vi "Get_Coeff_Fr_String.vi"(4 "String Name":string, 5 "Take New Data?":bool, 6 "Prefix":string, 7 "Show Dialog?":bool=TRUE, 8 "Sub String":string, 9 "Inst type":T1=enum."Raw voltage", 10 "Whole String":string) -> (0 "Coefficients Found?":bool, 2 "Calib Constants":dbl[](array[numeric]))   [LabVIEW 2010]
uses:
  Controls/Pressure_Units.ctl
  Controls/Inst_type.ctl
panel:
  in  "Pressure Units":T2
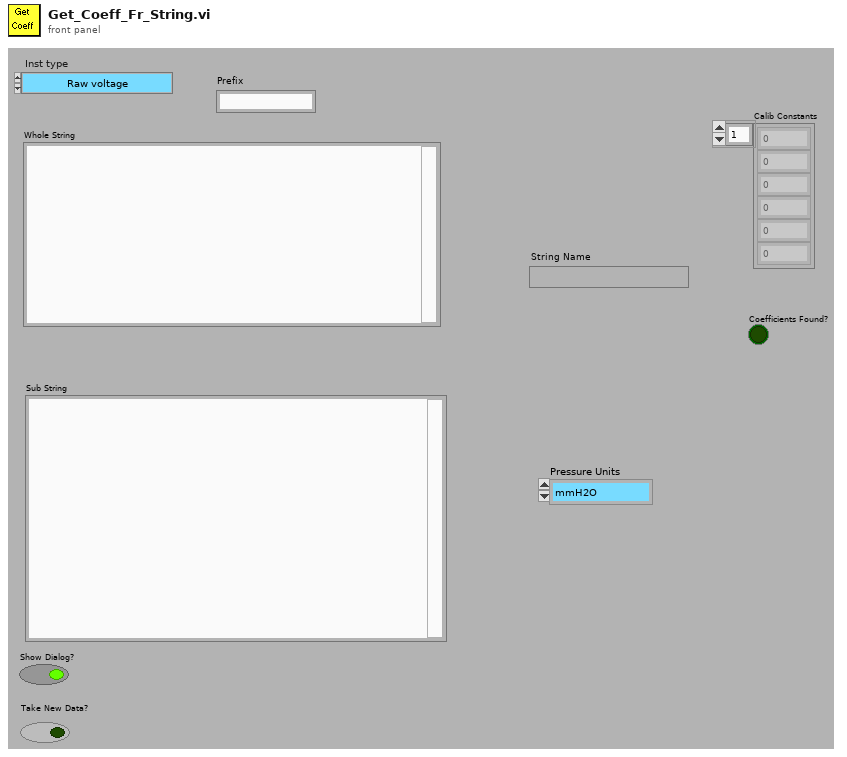
[diagram p1: front panel]
types:
  T1 = typedef "Inst_type.ctl" = enum16{"Propeller anemometer", "Raw voltage", "Pressure Transducer", "Pitot-static tube", "Preston tube", "Hot wire", "Cross wire 1", "Cross wire 2", "Generic Linear", "Generic Polynomial", "Generic BackPoly", "Fast FID", "Thermocouple", "Cold wire", "Pulsed Wire", "LDA Vel", "LDA Tran time", "LDA Arr time"}
  T2 = typedef "Pressure_Units.ctl" = enum16{"mmH2O", "mmHg", "Pa (N/m^2)", "mbar", "bar"}
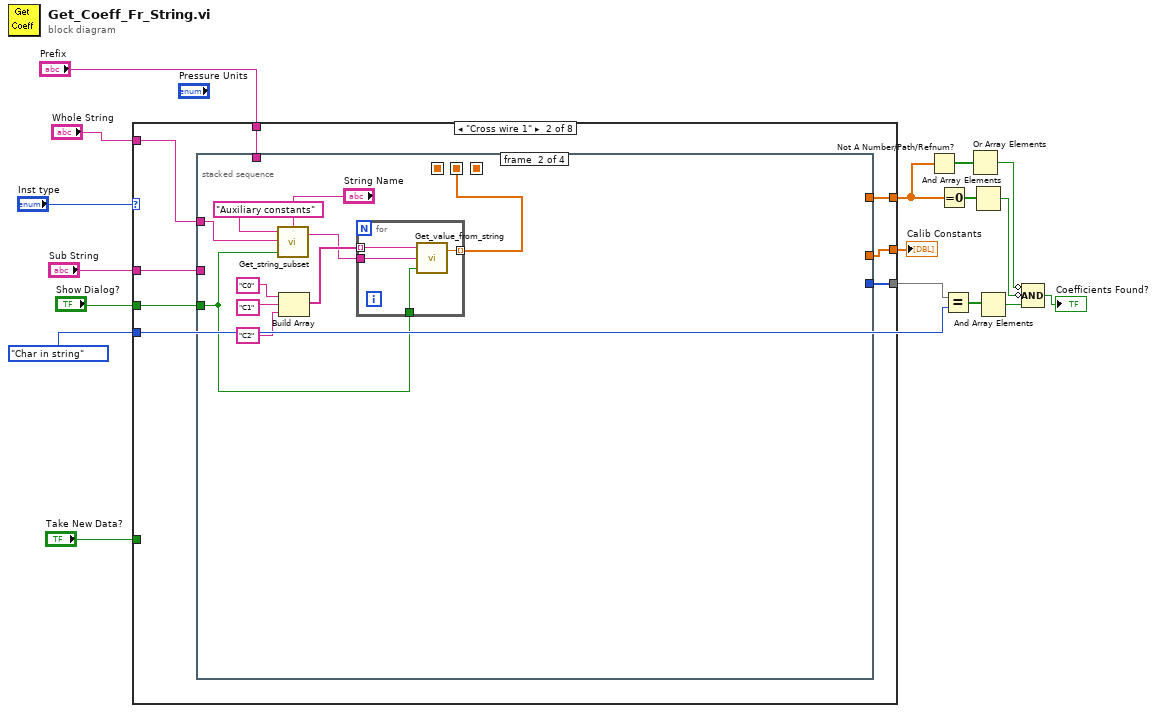
[diagram p0: block diagram]
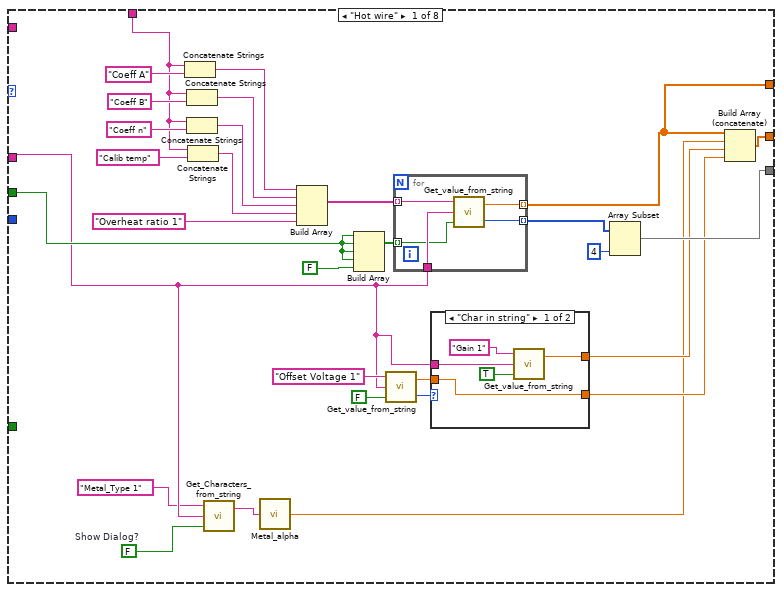
[diagram p2: hidden frame]
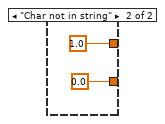
[diagram p3: hidden frame]
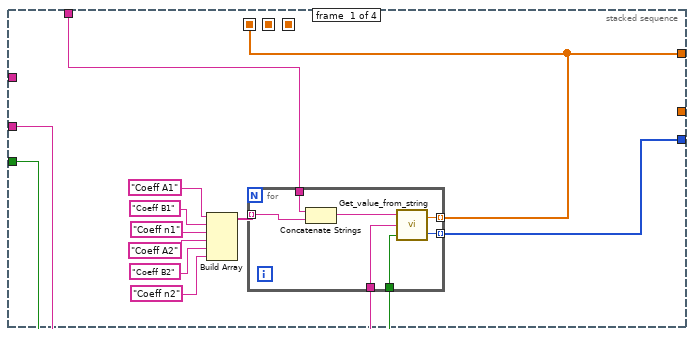
[diagram p4: hidden frame]
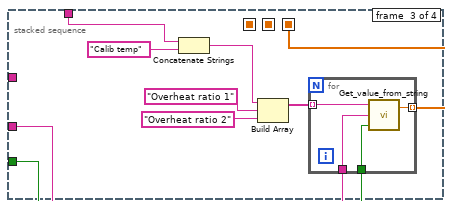
[diagram p5: hidden frame]
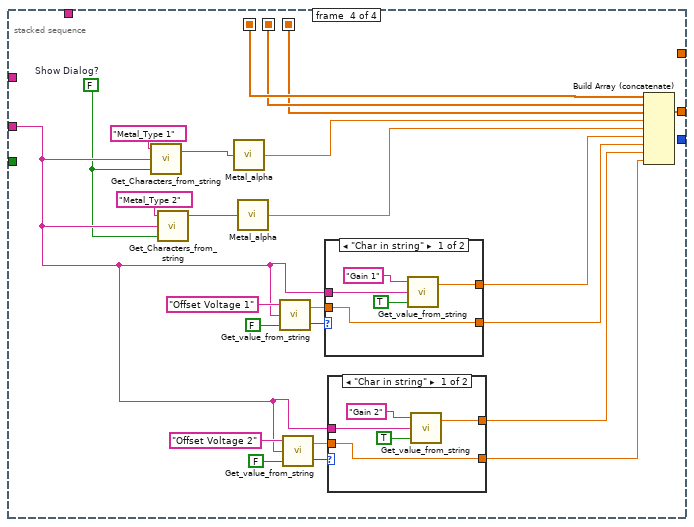
[diagram p6: hidden frame]
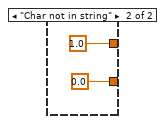
[diagram p7: hidden frame]
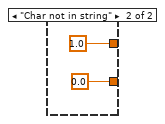
[diagram p8: hidden frame]
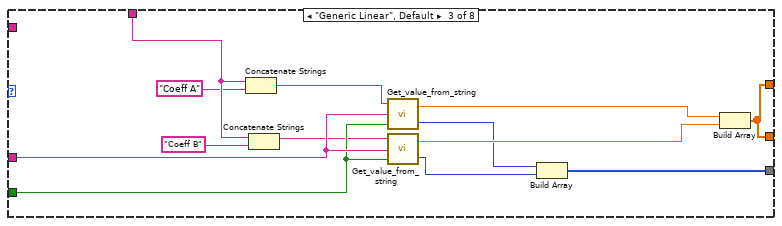
[diagram p9: hidden frame]
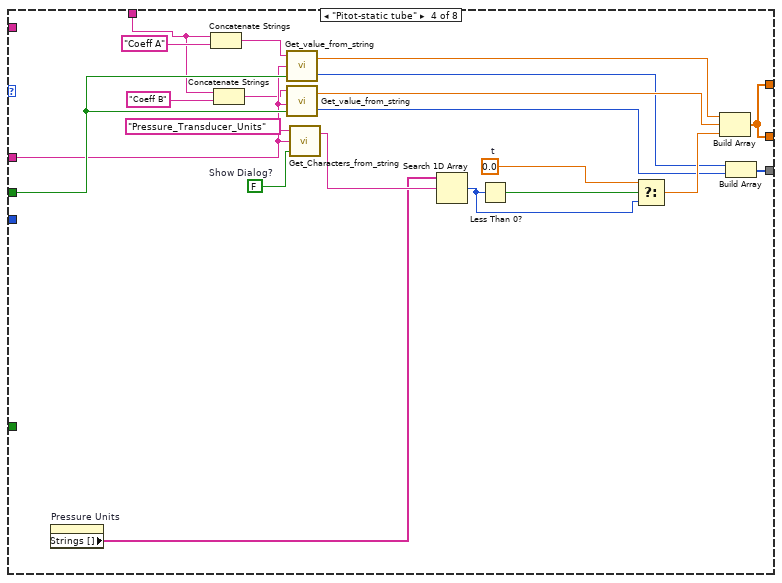
[diagram p10: hidden frame]
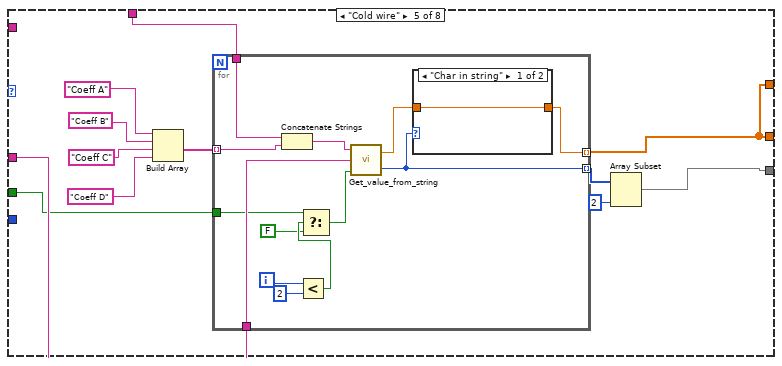
[diagram p11: hidden frame]
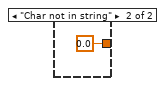
[diagram p12: hidden frame]
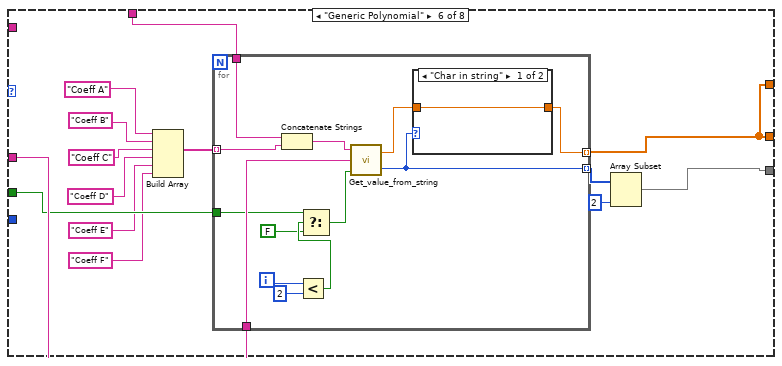
[diagram p13: hidden frame]
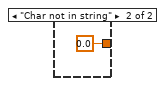
[diagram p14: hidden frame]
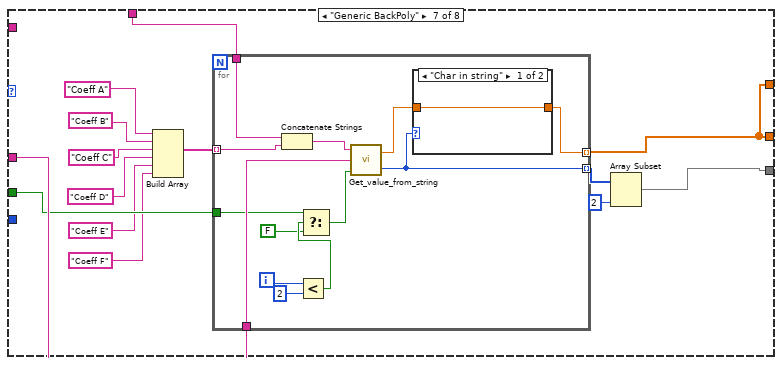
[diagram p15: hidden frame]
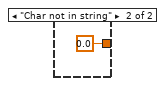
[diagram p16: hidden frame]
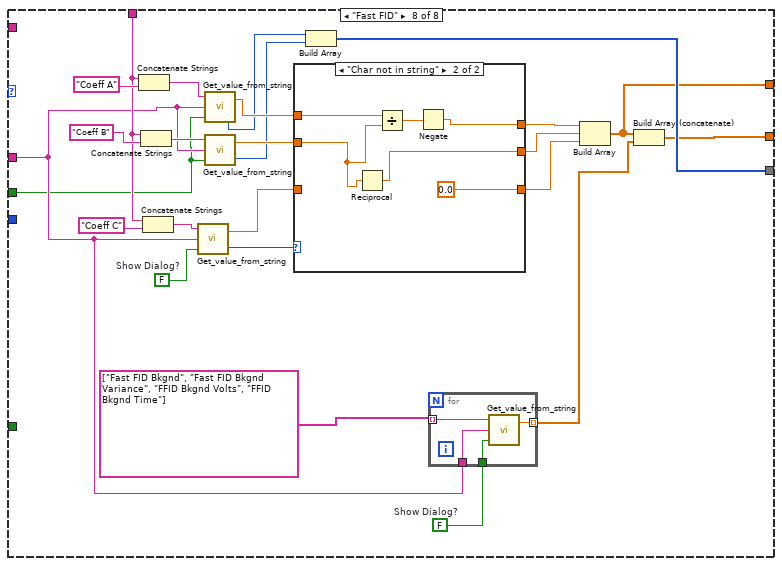
[diagram p17: hidden frame]
diagram:
  w8 = enum16{"Char in string", "Char not in string"}."Char in string" ("Status")
  n1 = case shown="\"Cross wire 1\"" "Inst type" {
    tunnel: [w47 w66 w151 w164 w185 w214 w243 w271] -> w14
    tunnel: "Sub String" -> [w25 w64 w161 w181 w191 w220 w249 w285]
    tunnel: "Whole String" -> [_ w65 _ _ _ _ _ _]
    tunnel: "Show Dialog?" -> [w29 w63 w160 w182 w189 w218 w247 w274]
    tunnel: "Prefix" -> [w37 w62 w159 w167 w190 w219 w248 w288]
    tunnel: "Take New Data?" -> [_ _ _ _ _ _ _ _]
    tunnel: [w30 w61 w152 w170 w186 w215 w244 w275] -> w10
    tunnel: w8 -> [_ _ _ _ _ _ _ _]
    tunnel: [w21 w60 w151 w164 w185 w214 w243 w270] -> w3
    frame "Hot wire" {
      w44 = FALSE  # Show Dialog?
      n2 = Concatenate Strings(w37, "Coeff A") -> (w33:string)
      n3 = Concatenate Strings(w37, "Coeff B") -> (w34:string)
      n4 = Concatenate Strings(w37, "Coeff n") -> (w35:string)
      n5 = Concatenate Strings(w37, "Calib temp") -> (w36:string)
      n6 = call "Get_Characters_from_string.vi"("Show Dialog?"=w44, "Input string"=w25, "Variable name"="Metal_Type 1") -> ("Value"=w19:string)  [unwired: 1 out]
      n7 = call "Metal_alpha.vi"("Metal_Type"=w19) -> ("alpha (/K)"=w18:dbl)
      n8 = Build Array(w33, w34, w35, w36, "Overheat ratio 1") -> (w45:string[])
      n9 = Build Array(w29, w29, w29, w29, FALSE ("Input Element")) -> (w42:bool[])
      n10 = call "Get_value_from_string.vi"("Show Dialog?"=FALSE, "Input string"=w25, "Variable name"="Offset Voltage 1") -> ("Status"=w26:enum16{"Char in string", "Char not in string"}, "Value"=w23:dbl)
      n11 = for {
        tunnel: w45 -> [w59] mode=indexing
        tunnel: w25 -> [w58]
        tunnel: [w57] -> w21 mode=indexing
        tunnel: w42 -> [w56] mode=indexing
        tunnel: [w55] -> w32 mode=indexing
        n12 = call "Get_value_from_string.vi"("Show Dialog?"=w56, "Input string"=w58, "Variable name"=w59) -> ("Status"=w55:enum16{"Char in string", "Char not in string"}, "Value"=w57:dbl)
      }
      n13 = case shown="\"Char in string\"" w26 {
        tunnel: w25 -> [w52 _]
        tunnel: [w49 1.0 ("Value")] -> w24
        tunnel: w23 -> [w48 _]
        tunnel: [w48 0.0 ("Value")] -> w22
        frame "Char in string" {
          n14 = call "Get_value_from_string.vi"("Show Dialog?"=TRUE, "Input string"=w52, "Variable name"="Gain 1") -> ("Value"=w49:dbl)  [unwired: 1 out]
        }
        frame "Char not in string" {
        }
      }
      n15 = Array Subset(array=w32, length=4) -> (w30:enum16{"Char in string", "Char not in string"}[])  [unwired: 1 in]
      n16 = Build Array (concatenate)(w21, w18, w24, w22) -> (w47:dbl[])
    }
    frame "Cross wire 1" {
      n17 = stacked-sequence {
        seq-local: [w67 _ _ _] -> [_ _ _ w133]
        seq-local: [_ w88 _ _] -> [_ _ _ w132]
        seq-local: [_ _ w105 _] -> [_ _ _ w131]
        tunnel: [_ _ _ w136] -> w66
        tunnel: w65 -> [_ w94 _ _]
        tunnel: w64 -> [w71 _ w107 w122]
        tunnel: w63 -> [w70 w87 w106 _]
        tunnel: w62 -> [w69 _ w100 _]
        tunnel: [w68 _ _ _] -> w61
        tunnel: [w67 _ _ _] -> w60
        frame #0 {
          n18 = Build Array("Coeff A1", "Coeff B1", "Coeff n1", "Coeff A2", "Coeff B2", "Coeff n2") -> (w72:string[])
          n19 = for {
            tunnel: w72 -> [w82] mode=indexing
            tunnel: w71 -> [w85]
            tunnel: [w84] -> w67 mode=indexing
            tunnel: w70 -> [w83]
            tunnel: w69 -> [w80]
            tunnel: [w79] -> w68 mode=indexing
            n20 = Concatenate Strings(w80, w82) -> (w81:string)
            n21 = call "Get_value_from_string.vi"("Show Dialog?"=w83, "Input string"=w85, "Variable name"=w81) -> ("Status"=w79:enum16{"Char in string", "Char not in string"}, "Value"=w84:dbl)
          }
        }
        frame #1 {
          n22 = call "Get_string_subset.vi"("String Name"="String Name", "Show Dialog?"=w87, "String to split"=w94, "File Label"="Auxiliary constants") -> ("Output string"=w89:string)  [unwired: 1 out]
          n23 = Build Array("C0", "C1", "C2") -> (w90:string[])
          n24 = for {
            tunnel: w90 -> [w99] mode=indexing
            tunnel: [w98] -> w88 mode=indexing
            tunnel: w87 -> [w97]
            tunnel: w89 -> [w96]
            n25 = call "Get_value_from_string.vi"("Show Dialog?"=w97, "Input string"=w96, "Variable name"=w99) -> ("Value"=w98:dbl)  [unwired: 1 out]
          }
        }
        frame #2 {
          n26 = Concatenate Strings(w100, "Calib temp") -> (w101:string)
          n27 = Build Array(w101, "Overheat ratio 1", "Overheat ratio 2") -> (w108:string[])
          n28 = for {
            tunnel: w108 -> [w112] mode=indexing
            tunnel: w107 -> [w111]
            tunnel: [w110] -> w105 mode=indexing
            tunnel: w106 -> [w109]
            n29 = call "Get_value_from_string.vi"("Show Dialog?"=w109, "Input string"=w111, "Variable name"=w112) -> ("Value"=w110:dbl)  [unwired: 1 out]
          }
        }
        frame #3 {
          w113 = FALSE  # Show Dialog?
          n30 = call "Get_Characters_from_string.vi"("Show Dialog?"=w113, "Input string"=w122, "Variable name"="Metal_Type 1") -> ("Value"=w116:string)  [unwired: 1 out]
          n31 = call "Get_Characters_from_string.vi"("Show Dialog?"=w113, "Input string"=w122, "Variable name"="Metal_Type 2") -> ("Value"=w117:string)  [unwired: 1 out]
          n32 = call "Metal_alpha.vi"("Metal_Type"=w116) -> ("alpha (/K)"=w115:dbl)
          n33 = call "Metal_alpha.vi"("Metal_Type"=w117) -> ("alpha (/K)"=w114:dbl)
          n34 = call "Get_value_from_string.vi"("Show Dialog?"=FALSE, "Input string"=w122, "Variable name"="Offset Voltage 1") -> ("Status"=w128:enum16{"Char in string", "Char not in string"}, "Value"=w127:dbl)
          n35 = call "Get_value_from_string.vi"("Show Dialog?"=FALSE, "Input string"=w122, "Variable name"="Offset Voltage 2") -> ("Status"=w125:enum16{"Char in string", "Char not in string"}, "Value"=w126:dbl)
          n36 = case shown="\"Char in string\"" w128 {
            tunnel: w122 -> [w148 _]
            tunnel: [w145 1.0 ("Value")] -> w121
            tunnel: w127 -> [w144 _]
            tunnel: [w144 0.0 ("Value")] -> w120
            frame "Char in string" {
              n37 = call "Get_value_from_string.vi"("Show Dialog?"=TRUE, "Input string"=w148, "Variable name"="Gain 1") -> ("Value"=w145:dbl)  [unwired: 1 out]
            }
            frame "Char not in string" {
            }
          }
          n38 = case shown="\"Char in string\"" w125 {
            tunnel: w122 -> [w141 _]
            tunnel: [w138 1.0 ("Value")] -> w118
            tunnel: w126 -> [w137 _]
            tunnel: [w137 0.0 ("Value")] -> w119
            frame "Char in string" {
              n39 = call "Get_value_from_string.vi"("Show Dialog?"=TRUE, "Input string"=w141, "Variable name"="Gain 2") -> ("Value"=w138:dbl)  [unwired: 1 out]
            }
            frame "Char not in string" {
            }
          }
          n40 = Build Array (concatenate)(w133, w132, w131, w115, w114, w121, w120, w118, w119) -> (w136:dbl[])
        }
      }
    }
    frame "Generic Linear", Default {
      n41 = Concatenate Strings(w159, "Coeff A") -> (w155:string)
      n42 = Concatenate Strings(w159, "Coeff B") -> (w156:string)
      n43 = call "Get_value_from_string.vi"("Show Dialog?"=w160, "Input string"=w161, "Variable name"=w155) -> ("Status"=w154:enum16{"Char in string", "Char not in string"}, "Value"=w162:dbl)
      n44 = call "Get_value_from_string.vi"("Show Dialog?"=w160, "Input string"=w161, "Variable name"=w156) -> ("Status"=w153:enum16{"Char in string", "Char not in string"}, "Value"=w163:dbl)
      n45 = Build Array(w154, w153) -> (w152:enum16{"Char in string", "Char not in string"}[])
      n46 = Build Array(w162, w163) -> (w151:dbl[])
    }
    frame "Pitot-static tube" {
      w175 = 0.0  # t
      w179 = FALSE  # Show Dialog?
      n47 = property on="Pressure Units" class="Enum (strict)"() -> ("Strings []"=w173:string[])  [unwired: 2 in, 2 out]
      n48 = Concatenate Strings(w167, "Coeff A") -> (w166:string)
      n49 = Concatenate Strings(w167, "Coeff B") -> (w165:string)
      n50 = call "Get_value_from_string.vi"("Show Dialog?"=w182, "Input string"=w181, "Variable name"=w166) -> ("Status"=w172:enum16{"Char in string", "Char not in string"}, "Value"=w183:dbl)
      n51 = call "Get_value_from_string.vi"("Show Dialog?"=w182, "Input string"=w181, "Variable name"=w165) -> ("Status"=w171:enum16{"Char in string", "Char not in string"}, "Value"=w184:dbl)
      n52 = call "Get_Characters_from_string.vi"("Show Dialog?"=w179, "Input string"=w181, "Variable name"="Pressure_Transducer_Units") -> ("Value"=w178:string)  [unwired: 1 out]
      n53 = Search 1D Array(1D array=w173, element=w178) -> (index of element=w176:i32)  [unwired: 1 out]
      n54 = Less Than 0?(x=w176) -> (x < 0?=w177:bool)
      n55 = Select(t=w175, s=w177, f=w176) -> (s? t:f=w174:dbl)
      n56 = Build Array(w183, w184, w174) -> (w164:dbl[])
      n57 = Build Array(w172, w171) -> (w170:enum16{"Char in string", "Char not in string"}[])
    }
    frame "Cold wire" {
      n58 = Build Array("Coeff A", "Coeff B", "Coeff C", "Coeff D") -> (w192:string[])
      n59 = for {
        tunnel: w192 -> [w208] mode=indexing
        tunnel: w191 -> [w209]
        tunnel: [w198] -> w185 mode=indexing
        tunnel: w190 -> [w207]
        tunnel: [w199] -> w187 mode=indexing
        tunnel: w189 -> [w202]
        i -> [w205]
        n60 = Concatenate Strings(w207, w208) -> (w206:string)
        n61 = Less?(x=w205, y=2) -> (x < y?=w203:bool)
        n62 = Select(t=w202, s=w203, f=FALSE) -> (s? t:f=w200:bool)
        n63 = call "Get_value_from_string.vi"("Show Dialog?"=w200, "Input string"=w209, "Variable name"=w206) -> ("Status"=w199:enum16{"Char in string", "Char not in string"}, "Value"=w197:dbl)
        n64 = case shown="\"Char in string\"" w199 {
          tunnel: [w210 0.0 ("Value")] -> w198
          tunnel: w197 -> [w210 _]
          frame "Char in string" {
          }
          frame "Char not in string" {
          }
        }
      }
      n65 = Array Subset(array=w187, length=2) -> (w186:enum16{"Char in string", "Char not in string"}[])  [unwired: 1 in]
    }
    frame "Generic Polynomial" {
      n66 = Build Array("Coeff A", "Coeff B", "Coeff C", "Coeff D", "Coeff E", "Coeff F") -> (w221:string[])
      n67 = for {
        tunnel: w221 -> [w237] mode=indexing
        tunnel: w220 -> [w238]
        tunnel: [w227] -> w214 mode=indexing
        tunnel: w219 -> [w236]
        tunnel: [w228] -> w216 mode=indexing
        tunnel: w218 -> [w231]
        i -> [w234]
        n68 = Concatenate Strings(w236, w237) -> (w235:string)
        n69 = Less?(x=w234, y=2) -> (x < y?=w232:bool)
        n70 = Select(t=w231, s=w232, f=FALSE) -> (s? t:f=w229:bool)
        n71 = call "Get_value_from_string.vi"("Show Dialog?"=w229, "Input string"=w238, "Variable name"=w235) -> ("Status"=w228:enum16{"Char in string", "Char not in string"}, "Value"=w226:dbl)
        n72 = case shown="\"Char in string\"" w228 {
          tunnel: [w239 0.0 ("Value")] -> w227
          tunnel: w226 -> [w239 _]
          frame "Char in string" {
          }
          frame "Char not in string" {
          }
        }
      }
      n73 = Array Subset(array=w216, length=2) -> (w215:enum16{"Char in string", "Char not in string"}[])  [unwired: 1 in]
    }
    frame "Generic BackPoly" {
      n74 = Build Array("Coeff A", "Coeff B", "Coeff C", "Coeff D", "Coeff E", "Coeff F") -> (w250:string[])
      n75 = for {
        tunnel: w250 -> [w266] mode=indexing
        tunnel: w249 -> [w267]
        tunnel: [w256] -> w243 mode=indexing
        tunnel: w248 -> [w265]
        tunnel: [w257] -> w245 mode=indexing
        tunnel: w247 -> [w260]
        i -> [w263]
        n76 = Concatenate Strings(w265, w266) -> (w264:string)
        n77 = Less?(x=w263, y=2) -> (x < y?=w261:bool)
        n78 = Select(t=w260, s=w261, f=FALSE) -> (s? t:f=w258:bool)
        n79 = call "Get_value_from_string.vi"("Show Dialog?"=w258, "Input string"=w267, "Variable name"=w264) -> ("Status"=w257:enum16{"Char in string", "Char not in string"}, "Value"=w255:dbl)
        n80 = case shown="\"Char in string\"" w257 {
          tunnel: [w268 0.0 ("Value")] -> w256
          tunnel: w255 -> [w268 _]
          frame "Char in string" {
          }
          frame "Char not in string" {
          }
        }
      }
      n81 = Array Subset(array=w245, length=2) -> (w244:enum16{"Char in string", "Char not in string"}[])  [unwired: 1 in]
    }
    frame "Fast FID" {
      w273 = FALSE  # Show Dialog?
      w294 = FALSE  # Show Dialog?
      n82 = Concatenate Strings(w288, "Coeff A") -> (w291:string)
      n83 = Concatenate Strings(w288, "Coeff B") -> (w289:string)
      n84 = Concatenate Strings(w288, "Coeff C") -> (w286:string)
      n85 = call "Get_value_from_string.vi"("Show Dialog?"=w294, "Input string"=w285, "Variable name"=w286) -> ("Status"=w293:enum16{"Char in string", "Char not in string"}, "Value"=w278:dbl)
      n86 = call "Get_value_from_string.vi"("Show Dialog?"=w274, "Input string"=w285, "Variable name"=w291) -> ("Status"=w277:enum16{"Char in string", "Char not in string"}, "Value"=w284:dbl)
      n87 = call "Get_value_from_string.vi"("Show Dialog?"=w274, "Input string"=w285, "Variable name"=w289) -> ("Status"=w276:enum16{"Char in string", "Char not in string"}, "Value"=w283:dbl)
      n88 = case shown="\"Char not in string\"" w293 {
        tunnel: w284 -> [w301 w306]
        tunnel: w283 -> [w300 w305]
        tunnel: [w301 w304] -> w282
        tunnel: [w300 w303] -> w281
        tunnel: [w299 0.0 ("new element/subarray")] -> w280
        tunnel: w278 -> [w299 _]
        frame "Char in string" {
        }
        frame "Char not in string" {
          n89 = Reciprocal(x=w305) -> (1/x=w303:dbl)
          n90 = Divide(x=w306, y=w305) -> (x/y=w307:dbl)
          n91 = Negate(x=w307) -> (-x=w304:dbl)
        }
      }
      n92 = Build Array(w277, w276) -> (w275:enum16{"Char in string", "Char not in string"}[])
      n93 = for {
        tunnel: string[] ["Fast FID Bkgnd", "Fast FID Bkgnd Variance", "FFID Bkgnd Volts", "FFID Bkgnd Time"] ("appended array") -> [w298] mode=indexing
        tunnel: w285 -> [w297]
        tunnel: [w296] -> w272 mode=indexing
        tunnel: w273 -> [w295]
        n94 = call "Get_value_from_string.vi"("Show Dialog?"=w295, "Input string"=w297, "Variable name"=w298) -> ("Value"=w296:dbl)  [unwired: 1 out]
      }
      n95 = Build Array(w282, w281, w280) -> (w270:dbl[])
      n96 = Build Array (concatenate)(w270, w272) -> (w271:dbl[])
    }
  }
  "Calib Constants" <- w14
  n97 = Not A Number/Path/Refnum?(number/path/refnum=w3) -> (NaN/Path/Refnum?=w2:bool[])
  n98 = Equal To 0?(x=w3) -> (x = 0?=w4:bool[])
  n99 = Equal?(x=w10, y=w8) -> (x = y?=w9:bool[])
  n100 = Or Array Elements(Boolean array=w2) -> (logical OR=w1:bool)
  n101 = And Array Elements(Boolean array=w4) -> (logical AND=w5:bool)
  n102 = And Array Elements(Boolean array=w9) -> (logical AND=w7:bool)
  n103 = Compound Arithmetic op=AND(invert w1, invert w5, w7) -> (→"Coefficients Found?":bool)
